vi "UDP Refresh Keys.vi"(8 "error in (no error)":errorcluster, 10 "UDP UI References":T2, 11 "node References":T1) -> (0 "error out":errorcluster, 2 "UDP UI References out":T2, 3 "node References out":T1)   [LabVIEW 2015, in "E2E Tag Exchange editor node.lvclass"]
uses:
  E2E Tag Exchange editor node.lvclass
  object references.ctl
  <vilib>/NI/DCAF/Tag Editor Core/Configuration Editor/Classes/Engine Parent/Engine Parent Editor Node.lvclass
  implementation specific/UDP/UDP UI References.ctl
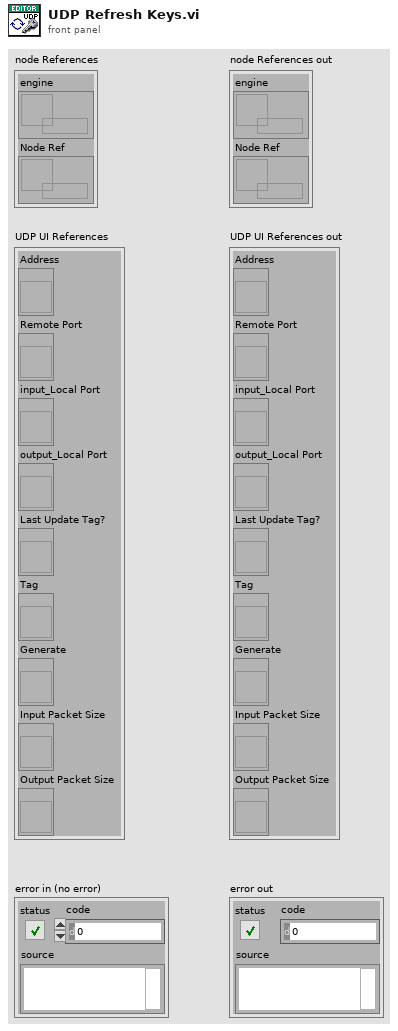
[diagram p1: front panel]
types:
  T1 = typedef "E2E Tag Exchange editor node.lvclass/object references.ctl" = cluster{"engine":refnum<data-value>, "Node Ref":refnum<data-value>}
  T2 = typedef "E2E Tag Exchange editor node.lvclass/UDP UI References.ctl" = cluster{"Address":refnum<vi>, "Remote Port":refnum<vi>, "input_Local Port":refnum<vi>, "output_Local Port":refnum<vi>, "Last Update Tag?":refnum<vi>, "Tag":refnum<vi>, "Generate":refnum<vi>, "Input Packet Size":refnum<vi>, "Output Packet Size":refnum<vi>}
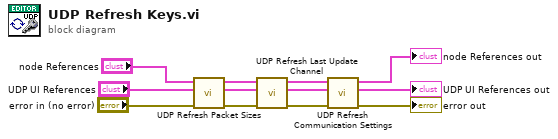
[diagram p0: block diagram]
diagram:
  n1 = call "UDP Refresh Packet Sizes.vi"("error in (no error)"="error in (no error)", "UDP UI References in"="UDP UI References", "node References"="node References") -> ("error out"=w1:errorcluster, "UDP UI References out"=w4:T2, "node References out"=w5:T1)  [unwired: 6 in]
  n2 = call "UDP Refresh Last Update Channel.vi"("error in (no error)"=w1, "UDP UI References in"=w4, "node References"=w5) -> ("error out"=w11:errorcluster, "UDP UI References out"=w10:T2, "node References out"=w9:T1)  [unwired: 6 in]
  n3 = call "UDP Refresh Communication Settings.vi"("error in (no error)"=w11, "UDP UI References"=w10, "node References"=w9) -> ("error out"=→"error out":errorcluster, "UDP UI References out"=→"UDP UI References out":T2, "node References out"=→"node References out":T1)  [unwired: 6 in]
